vi "readLUT.vi"(8 "error in (no error)":errorcluster, 11 "AOTF in":refnum<class "AOTF.lvclass">) -> (0 "error out":errorcluster, 3 "AOTF out":refnum<class "AOTF.lvclass">)   [LabVIEW 2012, in "AOTF.lvclass"]
uses:
  AOTF.lvclass
  Controls/MaxPower cluster.ctl
  Controls/LUT cluster.ctl
  AOTF.lvclass/AOTF.ctl
  <vilib>/Utility/file.llb/Read From Spreadsheet File (DBL).vi
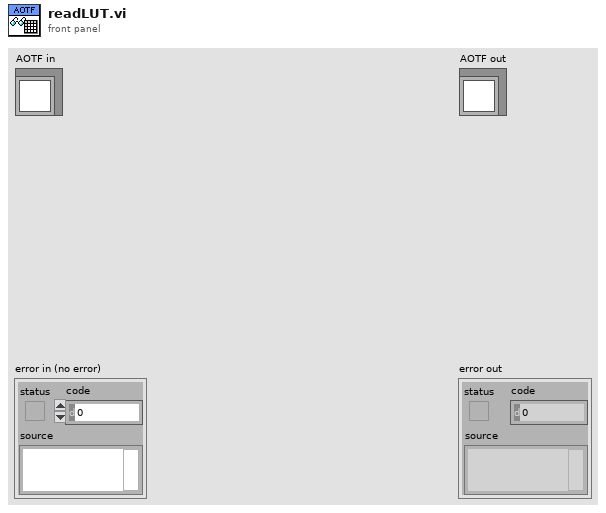
[diagram p1: front panel]
types:
  T1 = typedef "LUT cluster.ctl" = cluster{"LUT Array":dbl[][][]}
  T2 = typedef "MaxPower cluster.ctl" = cluster{"MaxPower Array":dbl[]}
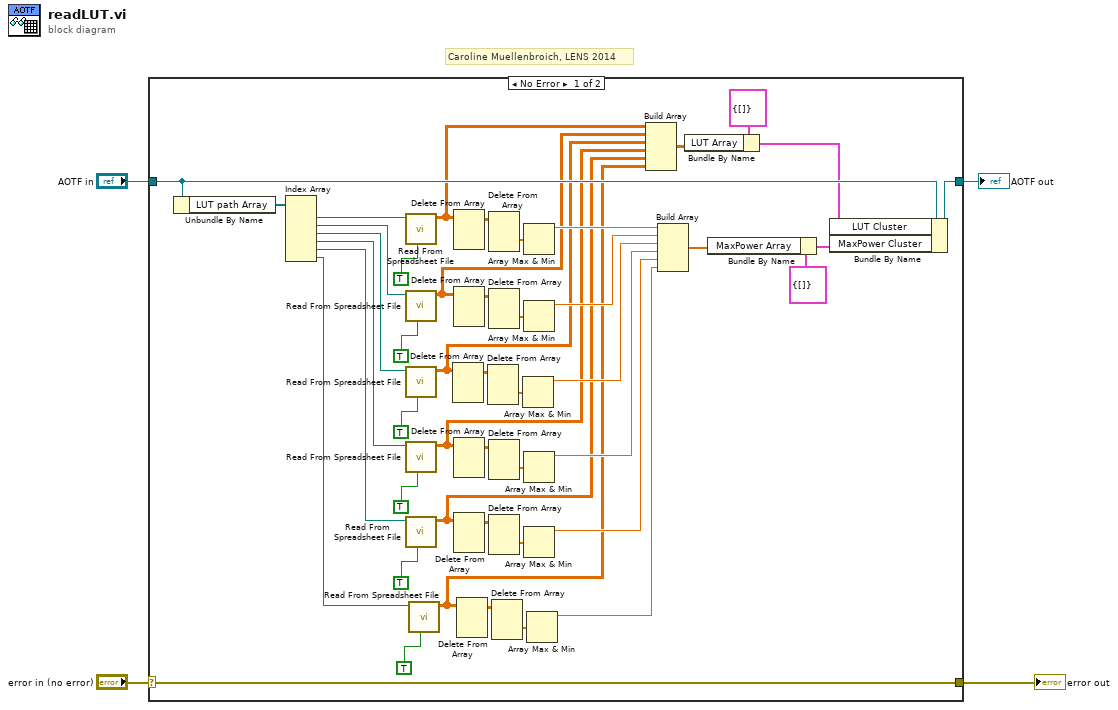
[diagram p0: block diagram]
diagram:
  # "Caroline Muellenbroich, LENS 2014"
  n1 = case shown="No Error" "error in (no error)" {
    selector: "error in (no error)" -> [w50 w52]
    tunnel: [w50 w52] -> w3
    tunnel: [w47 w51] -> w1
    tunnel: "AOTF in" -> [w48 w51]
    frame No Error {
      n2 = Unbundle By Name(w48) -> ("LUT path Array"=w44:path[])
      n3 = Index Array(array=w44) -> (element #1=w43:path, element #2=w30:path, element #3=w29:path, element #4=w28:path, element #5=w27:path, element #6=w7:path)  [unwired: 6 in]
      n4 = call-poly <vilib>:"Read From Spreadsheet File.vi"("transpose (no:F)"=TRUE, "file path (dialog if empty)"=w43) -> ("all rows"=w18:dbl[][])  [unwired: 5 in, 4 out]
      n5 = call-poly <vilib>:"Read From Spreadsheet File.vi"("transpose (no:F)"=TRUE, "file path (dialog if empty)"=w30) -> ("all rows"=w17:dbl[][])  [unwired: 5 in, 4 out]
      n6 = call-poly <vilib>:"Read From Spreadsheet File.vi"("transpose (no:F)"=TRUE, "file path (dialog if empty)"=w29) -> ("all rows"=w14:dbl[][])  [unwired: 5 in, 4 out]
      n7 = call-poly <vilib>:"Read From Spreadsheet File.vi"("transpose (no:F)"=TRUE, "file path (dialog if empty)"=w28) -> ("all rows"=w13:dbl[][])  [unwired: 5 in, 4 out]
      n8 = call-poly <vilib>:"Read From Spreadsheet File.vi"("transpose (no:F)"=TRUE, "file path (dialog if empty)"=w27) -> ("all rows"=w12:dbl[][])  [unwired: 5 in, 4 out]
      n9 = call-poly <vilib>:"Read From Spreadsheet File.vi"("transpose (no:F)"=TRUE, "file path (dialog if empty)"=w7) -> ("all rows"=w6:dbl[][])  [unwired: 5 in, 4 out]
      n10 = Delete From Array(array=w14) -> (array with subset deleted=w35:dbl[][])  [unwired: 3 in, 1 out]
      n11 = Delete From Array(array=w18) -> (array with subset deleted=w46:dbl[][])  [unwired: 3 in, 1 out]
      n12 = Delete From Array(array=w17) -> (array with subset deleted=w38:dbl[][])  [unwired: 3 in, 1 out]
      n13 = Delete From Array(array=w13) -> (array with subset deleted=w41:dbl[][])  [unwired: 3 in, 1 out]
      n14 = Delete From Array(array=w12) -> (array with subset deleted=w32:dbl[][])  [unwired: 3 in, 1 out]
      n15 = Delete From Array(array=w6) -> (array with subset deleted=w9:dbl[][])  [unwired: 3 in, 1 out]
      n16 = Delete From Array(array=w35) -> (deleted portion=w36:dbl[])  [unwired: 3 in, 1 out]
      n17 = Delete From Array(array=w46) -> (deleted portion=w45:dbl[])  [unwired: 3 in, 1 out]
      n18 = Delete From Array(array=w38) -> (deleted portion=w37:dbl[])  [unwired: 3 in, 1 out]
      n19 = Delete From Array(array=w41) -> (deleted portion=w42:dbl[])  [unwired: 3 in, 1 out]
      n20 = Delete From Array(array=w32) -> (deleted portion=w31:dbl[])  [unwired: 3 in, 1 out]
      n21 = Delete From Array(array=w9) -> (deleted portion=w8:dbl[])  [unwired: 3 in, 1 out]
      n22 = Array Max & Min(array=w36) -> (max value=w24:dbl)  [unwired: 3 out]
      n23 = Array Max & Min(array=w45) -> (max value=w26:dbl)  [unwired: 3 out]
      n24 = Array Max & Min(array=w37) -> (max value=w25:dbl)  [unwired: 3 out]
      n25 = Array Max & Min(array=w42) -> (max value=w23:dbl)  [unwired: 3 out]
      n26 = Array Max & Min(array=w31) -> (max value=w22:dbl)  [unwired: 3 out]
      n27 = Array Max & Min(array=w8) -> (max value=w5:dbl)  [unwired: 3 out]
      n28 = Build Array(w18, w17, w14, w13, w12, w6) -> (w16:dbl[][][])
      n29 = Build Array(w26, w25, w24, w23, w22, w5) -> (w21:dbl[])
      n30 = Bundle By Name(cluster=T1 {"LUT Array"=[]} ("LUT Cluster"), "LUT Array"=w16) -> (w15:T1)
      n31 = Bundle By Name(cluster=T2 {"MaxPower Array"=[]} ("MaxPower Cluster"), "MaxPower Array"=w21) -> (w19:T2)
      n32 = Bundle By Name(cluster=w48, "LUT Cluster"=w15, "MaxPower Cluster"=w19) -> (w47:refnum<class "AOTF.lvclass">)
    }
    frame Error {
    }
  }
  "error out" <- w3
  "AOTF out" <- w1
